vi "LINC Get Bit Stream.vi"(8 "bit size":i32, 9 "bit offset":i32, 10 "little endian":bool, 11 "data in":string) -> (2 "bytes":i32, 3 "data out":string)   [LabVIEW 2018, in "STEPkgDriver_LINC.lvlib"]
uses:
  STEPkgDriver_LINC.lvlib
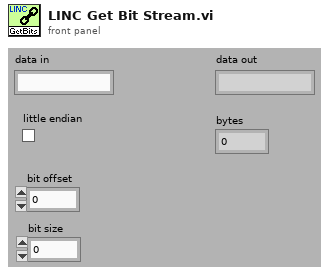
[diagram p1: front panel]
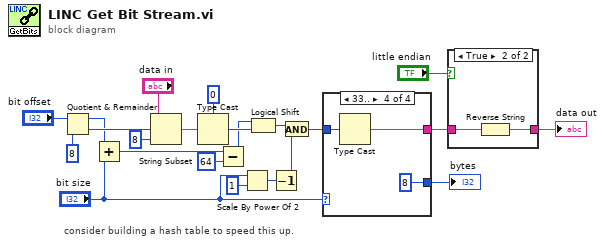
[diagram p0: block diagram]
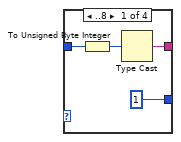
[diagram p3: hidden frame]
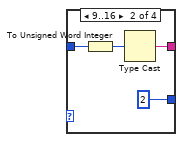
[diagram p4: hidden frame]
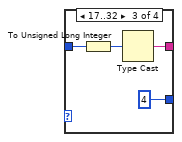
[diagram p5: hidden frame]
diagram:
  # "consider building a hash table to speed this up."
  n1 = Quotient & Remainder(x="bit offset", y=8) -> (x-y*floor(x/y)=w17:i32, floor(x/y)=w21:i32)
  n2 = Add(x=w17, y="bit size") -> (x+y=w15:i32)
  n3 = String Subset(string="data in", offset (0)=w21, length (rest)=8 ("length (rest)")) -> (substring=w16:string)
  n4 = Type Cast(type=u64 0, x=w16) -> (*(type *) &x=w13:u64)
  n5 = Subtract(x=w15, y=64) -> (x-y=w7:i32)
  n6 = Scale By Power Of 2(n="bit size", x=u64 1) -> (x*2^n=w9:u64)
  n7 = Logical Shift(y=w7, x=w13) -> (x << y=w11:u64)
  n8 = Decrement(x=w9) -> (x-1=w8:u64)
  n9 = And(x=w11, y=w8) -> (x .and. y?=w6:u64)
  n10 = case shown="33.." "bit size" {
    tunnel: [w25 w29 w33 w37] -> w3
    tunnel: w6 -> [w24 w28 w32 w36]
    tunnel: [1 2 4 8] -> w1
    frame ..8 {
      n11 = To Unsigned Byte Integer(number=w24) -> (unsigned 8bit integer=w26:u8)
      n12 = Type Cast(x=w26) -> (*(type *) &x=w25:string)  [unwired: 1 in]
    }
    frame 9..16 {
      n13 = To Unsigned Word Integer(number=w28) -> (unsigned 16bit integer=w30:u16)
      n14 = Type Cast(x=w30) -> (*(type *) &x=w29:string)  [unwired: 1 in]
    }
    frame 17..32 {
      n15 = To Unsigned Long Integer(number=w32) -> (unsigned 32bit integer=w34:u32)
      n16 = Type Cast(x=w34) -> (*(type *) &x=w33:string)  [unwired: 1 in]
    }
    frame 33.. {
      n17 = Type Cast(x=w36) -> (*(type *) &x=w37:string)  [unwired: 1 in]
    }
  }
  "bytes" <- w1
  n18 = case shown="True" "little endian" {
    tunnel: w3 -> [w38 w40]
    tunnel: [w38 w39] -> w2
    frame False {
    }
    frame True {
      n19 = Reverse String(1:w40) -> (0:w39:string)
    }
  }
  "data out" <- w2
